vi "Panel Fader.vi"(0 "Vi reference":refnum<vi>, 1 "Transparent FP Effect? (F)":bool, 7 "Fade Speed  (ms per % change)":u32=5, 11 "error in (no error)":errorcluster, 12 "Fade Direction (Fade Out)":enum16{"Fade Out", "Fade In"}(ring)) -> (4 "Vi reference out":refnum<vi>, 15 "error out":errorcluster)   [LabVIEW 2014, in "Endigit.lvlib"]
doc: "Panel Fader.vi\n\nThis VI fades the front panel of the VI specified by the Vi reference control in or out depending on the setting of the Fade Out / In control. The user can specify the fade speed by setting the Fade Speed control. The fade speed is specified in milliseconds per % change.\n\nIf the VI specified by the Vi reference control is utilizing a transparent front Panel effect, set the Transparent FP Effect? input true. This prevents the front panel transparency attribute from being manipulated during the fade out operation. If the front panel transparency attribute is manipulated during the fade out operation, the transparent FP effect is ended.\n\nInputs:\nVI reference - Reference to the VI to operate on.\n\nFade Direction (Fade Out) - Specifies the fade direction (out (default) or in).\n\nFade Speed (ms per % change) - Sets the fade speed (ms per % change).\n\nTransparent FP Effect? (F) - Indicates that the VI being acted upon utilizes the transparent FP effect.\n\nerror in - Standard error cluster.\n\nOutputs:\nVI reference - Reference to the VI to operate on.\n\nerror out - Standard error cluster.\n\nDeveloped By:\nMark Ridgley\nMark.Ridgley_LabVIEW.Developer@comcast.net"
uses:
  Endigit.lvlib
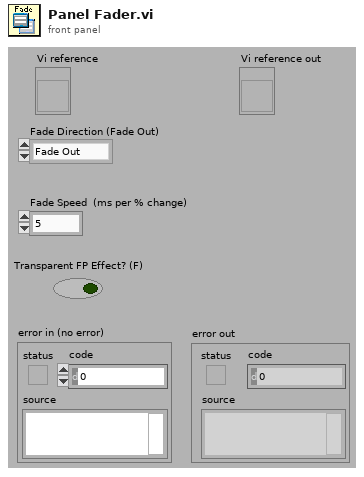
[diagram p1: front panel]
types:
  T1 = enum32{"Invalid", "Standard", "Closed", "Hidden", "Minimized", "Maximized"}
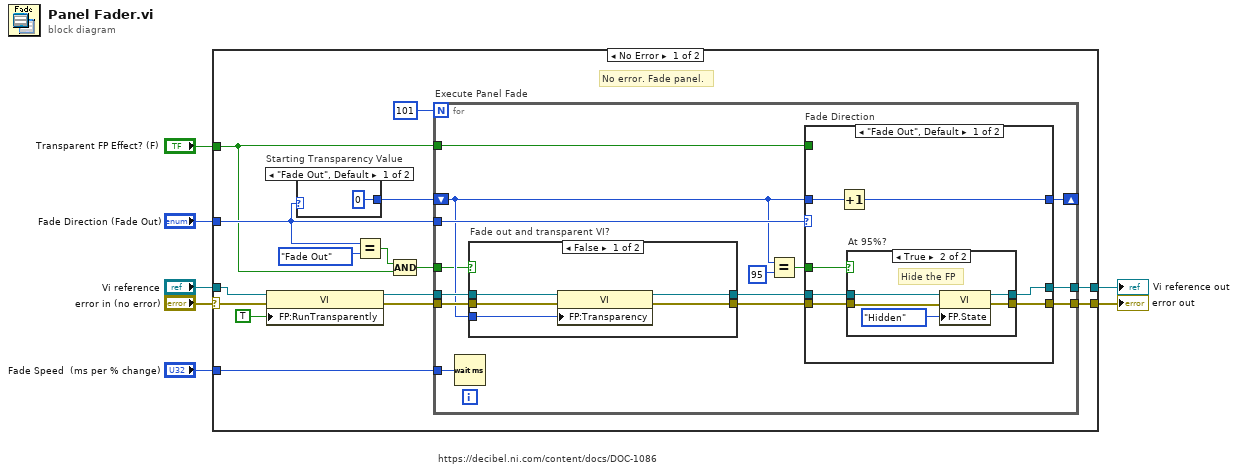
[diagram p0: block diagram]
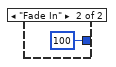
[diagram p2: hidden frame]
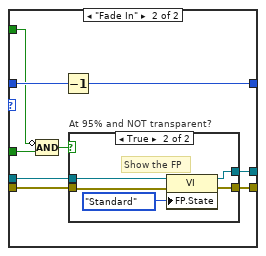
[diagram p5: hidden frame]
diagram:
  # "https://decibel.ni.com/content/docs/DOC-1086"
  n1 = case shown="No Error" "error in (no error)" {
    selector: "error in (no error)" -> [w13 w77]
    tunnel: "Fade Speed  (ms per % change)" -> [w21 _]
    tunnel: "Fade Direction (Fade Out)" -> [w12 _]
    tunnel: "Vi reference" -> [w17 w76]
    tunnel: [w15 w77] -> w4
    tunnel: [w14 w76] -> w3
    tunnel: "Transparent FP Effect? (F)" -> [w8 _]
    frame No Error {
      # "No error. Fade panel."
      n2 = property class="VI"(reference=w17, error in=w13, "FP:RunTransparently"=TRUE ("Front Panel Window:Run VI Transparently")) -> (reference out=w18:refnum<vi>, error out=w19:errorcluster)
      n3 = case "Starting Transparency Value" shown="\"Fade Out\", Default" w12 {
        tunnel: [u8 0 ("t") u8 100 ("t")] -> w20
        frame "Fade Out", Default {
        }
        frame "Fade In" {
        }
      }
      n4 = Equal?(x=w12, y=enum16{"Fade Out", "Fade In"}."Fade Out") -> (x = y?=w10:bool)
      n5 = Compound Arithmetic op=AND(w10, w8) -> (w9:bool)
      n6 = for "Execute Panel Fade" {
        N: 101 -> [_]
        tunnel: w18 -> [w38]
        tunnel: w19 -> [w37]
        shift-right: [w36] -> _
        shift-left: w20 -> [w27]
        tunnel: w12 -> [w35]
        tunnel: w21 -> [w34]
        tunnel: [w31] -> w15
        tunnel: [w30] -> w14
        tunnel: w9 -> [w26]
        tunnel: w8 -> [w25]
        n7 = Wait (ms)(milliseconds to wait=w34) -> ()  [unwired: 1 out]
        n8 = case "Fade out and transparent VI?" shown="False" w26 {
          tunnel: w38 -> [w43 w45]
          tunnel: w37 -> [w42 w44]
          tunnel: [w41 w44] -> w33
          tunnel: [w40 w45] -> w32
          tunnel: w27 -> [w39 _]
          frame False {
            n9 = property class="VI"(reference=w43, error in=w42, "FP:Transparency"=w39) -> (reference out=w40:refnum<vi>, error out=w41:errorcluster)
          }
          frame True {
            # "Do not set FP transparency because doing so ends the transparent VI effect."
          }
        }
        n10 = Equal?(x=w27, y=u8 95) -> (x = y?=w28:bool)
        n11 = case "Fade Direction" shown="\"Fade Out\", Default" w35 {
          tunnel: w27 -> [w52 w68]
          tunnel: [w51 w67] -> w36
          tunnel: [w47 w66] -> w30
          tunnel: [w49 w65] -> w31
          tunnel: w33 -> [w50 w64]
          tunnel: w32 -> [w48 w63]
          tunnel: w28 -> [w46 w62]
          tunnel: w25 -> [_ w60]
          frame "Fade Out", Default {
            n12 = Increment(x=w52) -> (x+1=w51:u8)
            n13 = case "At 95%?" shown="True" w46 {
              tunnel: w48 -> [w54 w58]
              tunnel: [w54 w57] -> w47
              tunnel: [w53 w56] -> w49
              tunnel: w50 -> [w53 w55]
              frame False {
              }
              frame True {
                # "Hide the FP"
                n14 = property class="VI"(reference=w58, error in=w55, "FP.State"=T1."Hidden" ("Front Panel Window:State")) -> (reference out=w57:refnum<vi>, error out=w56:errorcluster)
              }
            }
          }
          frame "Fade In" {
            n15 = Compound Arithmetic op=AND(invert w60, w62) -> (w61:bool)
            n16 = Decrement(x=w68) -> (x-1=w67:u8)
            n17 = case "At 95% and NOT transparent?" shown="True" w61 {
              tunnel: w63 -> [w70 w74]
              tunnel: [w70 w73] -> w66
              tunnel: [w69 w72] -> w65
              tunnel: w64 -> [w69 w71]
              frame False {
              }
              frame True {
                # "Show the FP"
                n18 = property class="VI"(reference=w74, error in=w71, "FP.State"=T1."Standard" ("Front Panel Window:State")) -> (reference out=w73:refnum<vi>, error out=w72:errorcluster)
              }
            }
          }
        }
      }
    }
    frame Error {
      # "Incoming error. Take no action."
    }
  }
  "error out" <- w4
  "Vi reference out" <- w3
